vi "Panel.vi"   [LabVIEW 2016, in "Rectangle Mask.lvclass"]
uses:
  Classes/Rectangle Mask/Rectangle Mask.lvclass
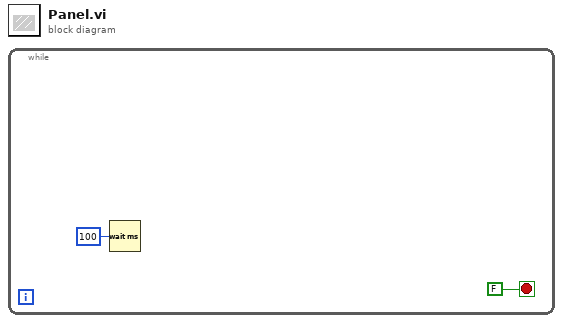
[diagram p0: block diagram]
diagram:
  n1 = while {
    stop <- FALSE stop-if-true
    n2 = Wait (ms)(milliseconds to wait=u32 100) -> ()  [unwired: 1 out]
  }
